vi "Add Generated Process to Project.vi"(8 "error in (no error)":errorcluster, 11 "Process Generator in":refnum<class "Process Generator.lvclass">) -> (0 "error out":errorcluster, 3 "Process Generator out":refnum<class "Process Generator.lvclass">)   [LabVIEW 2020, in "Process Generation.lvlib" / "Process Generator.lvclass"]
uses:
  Process Generator.lvclass
  Process Generator.lvclass/Process Generator.ctl
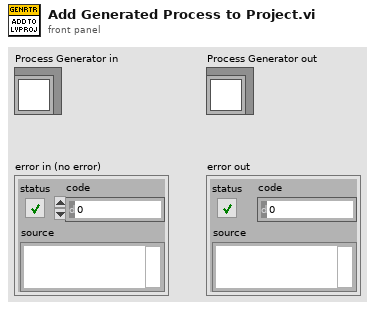
[diagram p1: front panel]
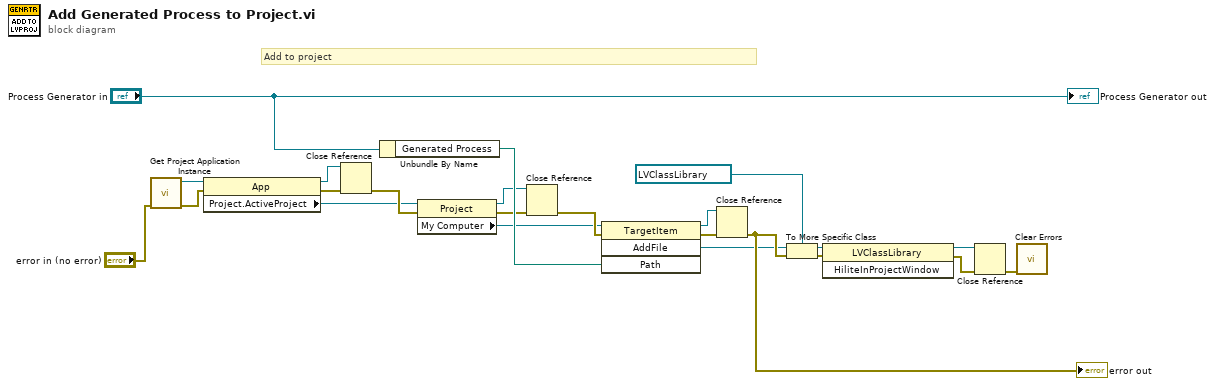
[diagram p0: block diagram]
diagram:
  # "Add to project"
  n1 = call "Get Project Application Instance.vi"("error in (no error)"="error in (no error)") -> ("error out"=w20:errorcluster, "Application out"=w19:refnum<vi>)  [unwired: 9 in]
  n2 = property class="App"(reference=w19, error in=w20) -> (reference out=w7:refnum<vi>, error out=w2:errorcluster, "Project.ActiveProject"=w1:refnum<vi>)
  n3 = Close Reference(reference=w7, error in (no error)=w2) -> (error out=w6:errorcluster)
  n4 = Unbundle By Name("Process Generator in") -> ("Generated Process"=w23:path)
  n5 = property class="Project"(reference=w1, error in=w6) -> (reference out=w9:refnum<vi>, error out=w4:errorcluster, "My Computer"=w3:refnum<vi>)
  n6 = Close Reference(reference=w9, error in (no error)=w4) -> (error out=w8:errorcluster)
  n7 = invoke class="TargetItem" method="AddFile"(reference=w3, error in=w8, "Path"=w23) -> (reference out=w10:refnum<vi>, error out=w5:errorcluster, "AddFile"=w13:refnum<vi>)  [unwired: 1 in, 1 out]
  n8 = Close Reference(reference=w10, error in (no error)=w5) -> (error out=w14:errorcluster)
  "error out" <- w14
  n9 = To More Specific Class(target class=refnum<vi> refnum ("reference"), reference=w13, error in=w14) -> (specific class reference=w11:refnum<vi>, error out=w15:errorcluster)
  n10 = invoke class="LVClassLibrary" method="HiliteInProjectWindow"(reference=w11, error in=w15) -> (reference out=w17:refnum<vi>, error out=w16:errorcluster)  [unwired: 1 in, 1 out]
  n11 = Close Reference(reference=w17, error in (no error)=w16) -> (error out=w18:errorcluster)
  n12 = call <vilib>:"Clear Errors.vi"("error in (no error)"=w18) -> ()  [unwired: 5 in, 2 out]
  "Process Generator out" <- "Process Generator in"
